vi "Initialise Timers.vi"(8 "error in (no error)":errorcluster, 11 "Main Controller in":refnum<class "Main Controller Actor.lvclass">) -> (0 "error out":errorcluster, 3 "Main Controller out":refnum<class "Main Controller Actor.lvclass">)   [LabVIEW 2021, in "Main Controller Actor.lvclass"]
uses:
  Main Controller Actor.lvclass
  Re-use Libraries/Vector 2D/Vector 2D.lvclass
  Task Scheduler/API/Task Scheduler Actor API.lvclass
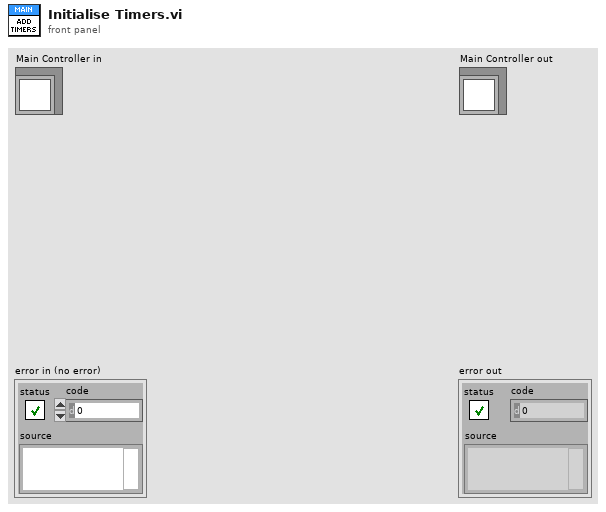
[diagram p1: front panel]
types:
  T1 = typedef "Constants.ctl" = cluster{"Colours":cluster{"OK":u32, "Warning":u32, "Error":u32, "Red":u32, "Green":u32, "Blue":u32, "Yellow":u32}, "System":cluster{"Target Frames Second":dbl, "World Size":T2, "Window Size":T2, "Battle Area Size":T2, "Sidebar Width":sgl, "SC2 Frame Rate [Seconds/Frame]":sgl, "Sidebar Player 2 Y Offset":sgl, "Windows Size V2":refnum<class "Vector 2D.lvclass">, "World Size V2":refnum<class "Vector 2D.lvclass">, "Battle Area Size V2":refnum<class "Vector 2D.lvclass">}, "Game":cluster{"Maximum Asteroids":i32, "Max Energy":i32, "Max Crew":i32, "Maximum Stars":i32}}
  T2 = typedef "SDL2 Utility.lvlib/Point (I32).ctl" = cluster{"x":i32, "y":i32}
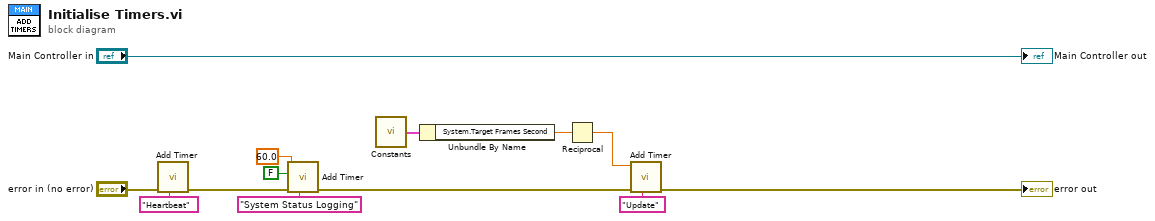
[diagram p0: block diagram]
diagram:
  n1 = call "Add Timer.vi"("Name"="Heartbeat", "error in (no error)"="error in (no error)") -> ("error out"=w11:errorcluster)  [unwired: 9 in]
  n2 = call "Add Timer.vi"("Name"="System Status Logging", "error in (no error)"=w11, "Enabled (T)"=FALSE, "Period (1) [s]"=60.0) -> ("error out"=w5:errorcluster)  [unwired: 7 in]
  n3 = call "Constants.vi"() -> ("Constants"=w3:T1)
  n4 = Unbundle By Name(w3) -> ("System.Target Frames Second"=w2:dbl)
  n5 = Reciprocal(x=w2) -> (1/x=w1:dbl)
  n6 = call "Add Timer.vi"("Name"="Update", "error in (no error)"=w5, "Period (1) [s]"=w1) -> ("error out"=→"error out":errorcluster)  [unwired: 8 in]
  "Main Controller out" <- "Main Controller in"
